vi "_PC_Pub_FM ctrlInstrRefNum.vi"(7 "function":T1, 8 "error in (no error)":errorcluster, 11 "Refnum":T2) -> (0 "error out":errorcluster)   [LabVIEW 2018]
uses:
  ctl/_PC_Pub_FM ctrlFileRefnumEnum.ctl
  Constant/AccessFolderName.ctl
  Ctl/RegistyFunc.ctl
  ctl/_PC_Pub_FM stateMachineEnum.ctl
  <vilib>/Utility/error.llb/Error Cluster From Error Code.vi
  <vilib>/ErrorRing/Error Ring.xnode
  FM.lvclass
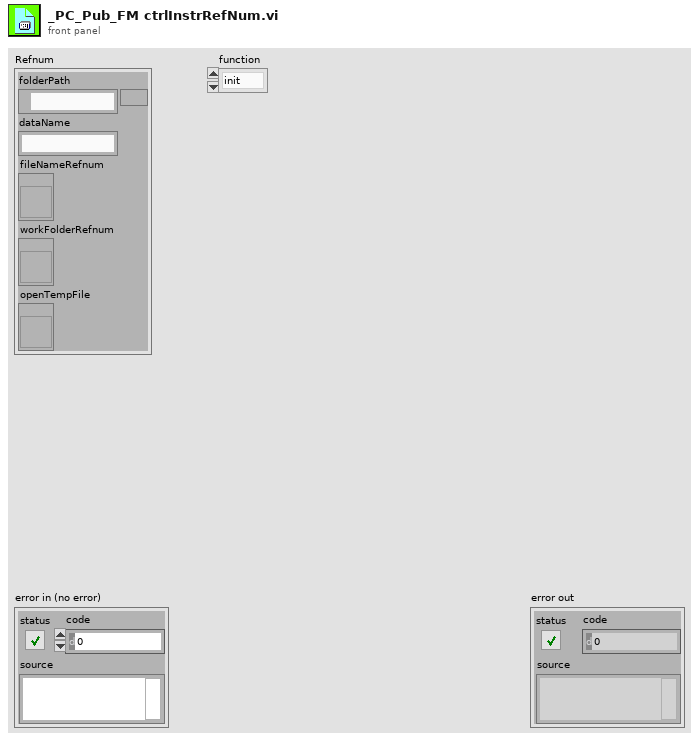
[diagram p1: front panel]
types:
  T1 = typedef "_PC_Pub_FM ctrlFileRefnumEnum.ctl" = enum16{"init", "checkFileName", "updFileName", "updWorkFolder", "updDataItems", "addNewFileName", "addSerialNum"}
  T2 = cluster{"folderPath":path, "dataName":string, "fileNameRefnum":refnum<vi>, "workFolderRefnum":refnum<vi>, "openTempFile":refnum<vi>}
  T3 = typedef "_PC_Pub_FM stateMachineEnum.ctl" = enum16{"none", "init", "reset_t0", "openTDMS", "writeTDMS", "closeTDMS", "readTDMS", "getDataItems"}
  T4 = typedef "RegistyFunc.ctl" = enum16{"None", "FileAutoSave", "FileNoise", "FileSN", "ExeStatu", "WorkFolderPath", "MethodPath", "AVGItem", "LoopItem", "AutoRun", "BGColor", "LineColor", "LineWidth", "XGrid", "YGrid", "DeviceRefnum"}
  T5 = typedef "AccessFolderName.ctl" = enum16{"None", "system_log", "ui_log", "msdata", "method", "d999_param"}
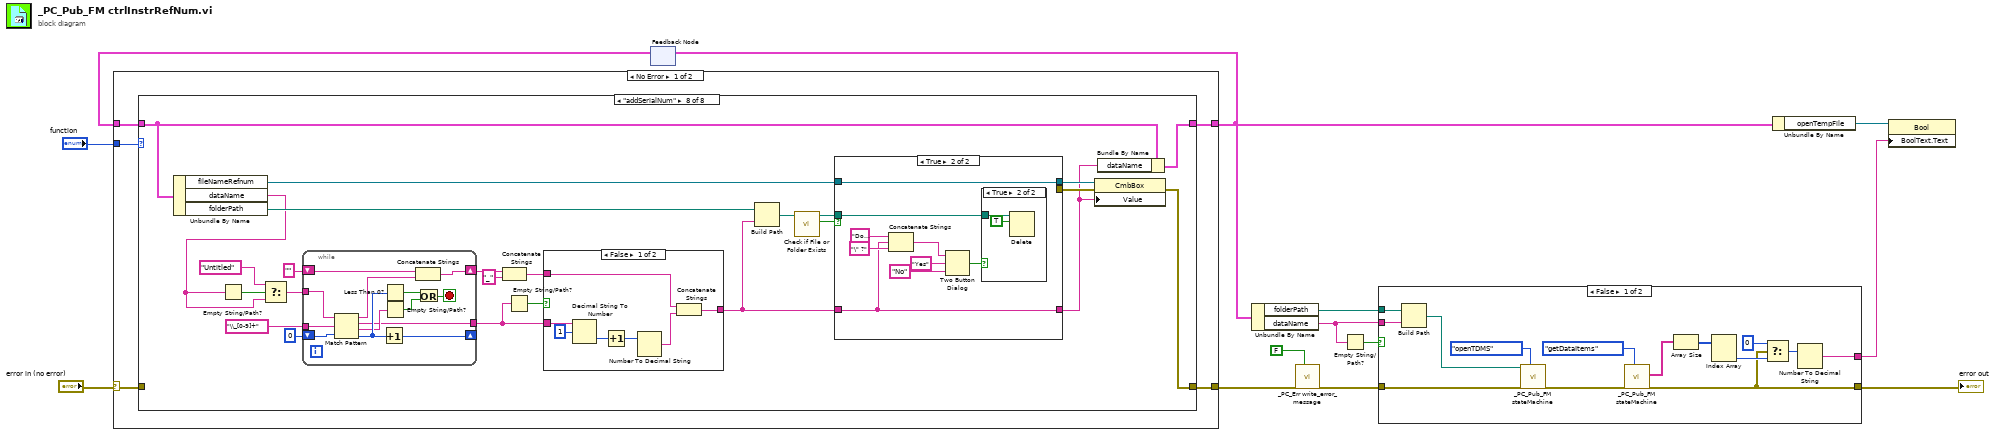
[diagram p0: block diagram]
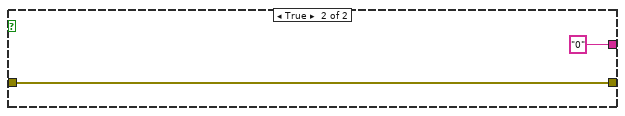
[diagram p2: hidden frame]
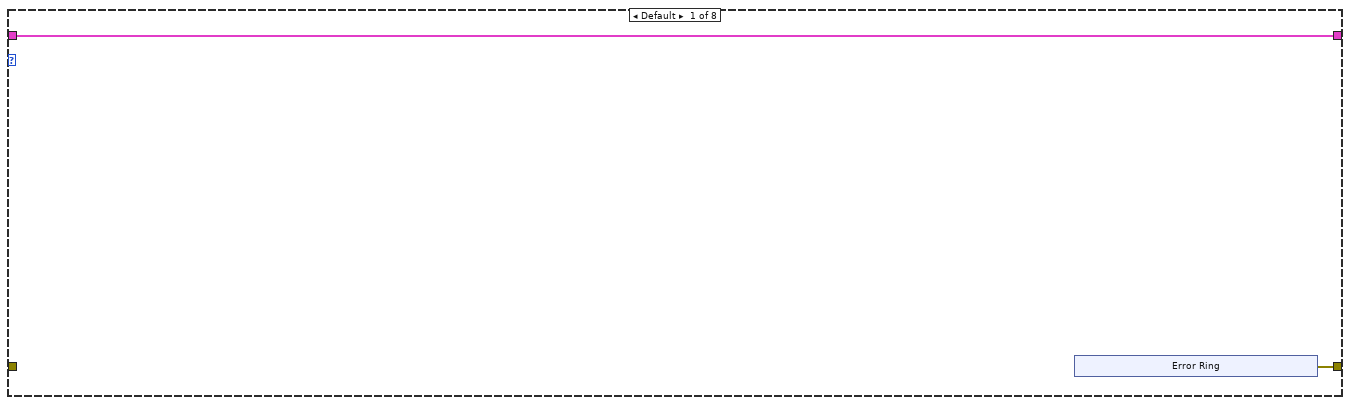
[diagram p3: hidden frame]
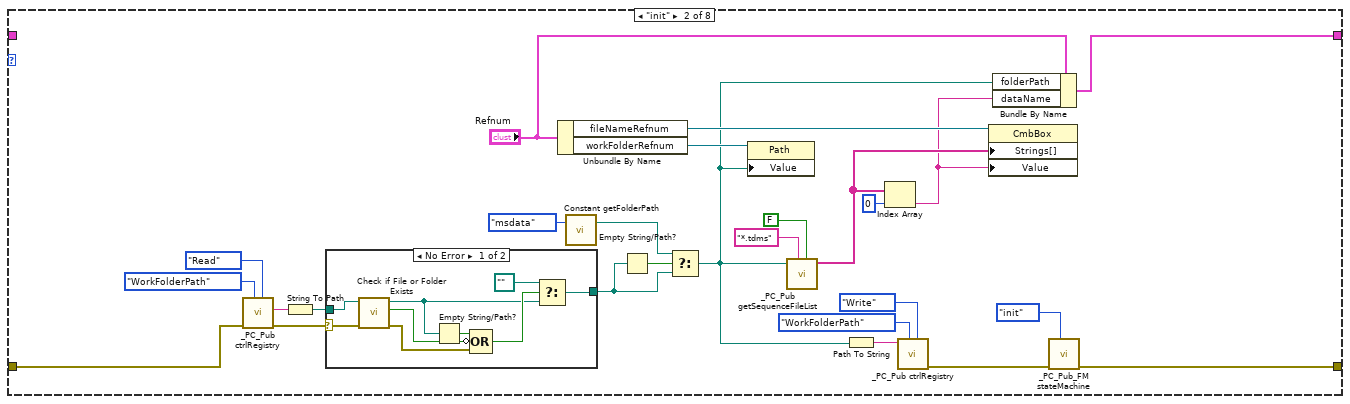
[diagram p4: hidden frame]
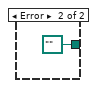
[diagram p5: hidden frame]
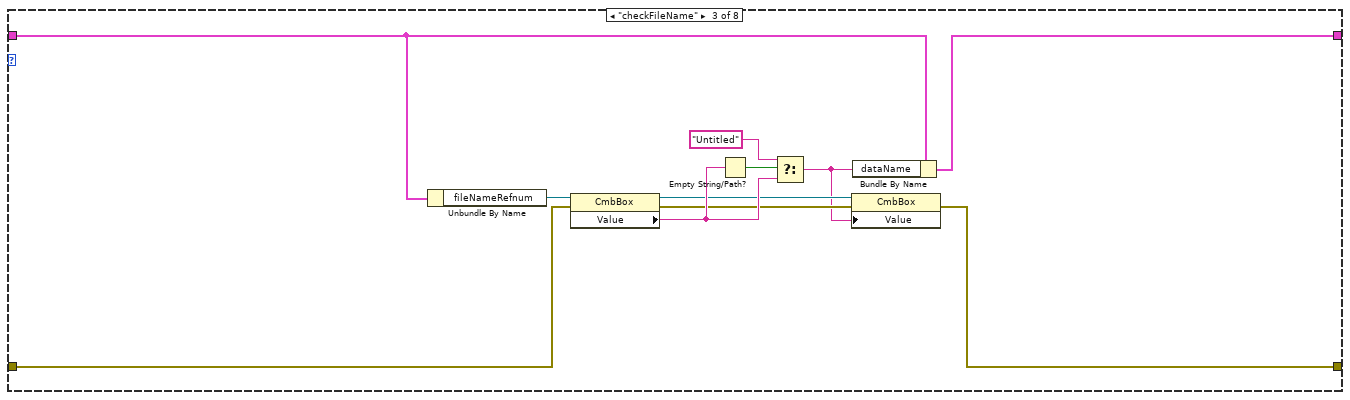
[diagram p6: hidden frame]
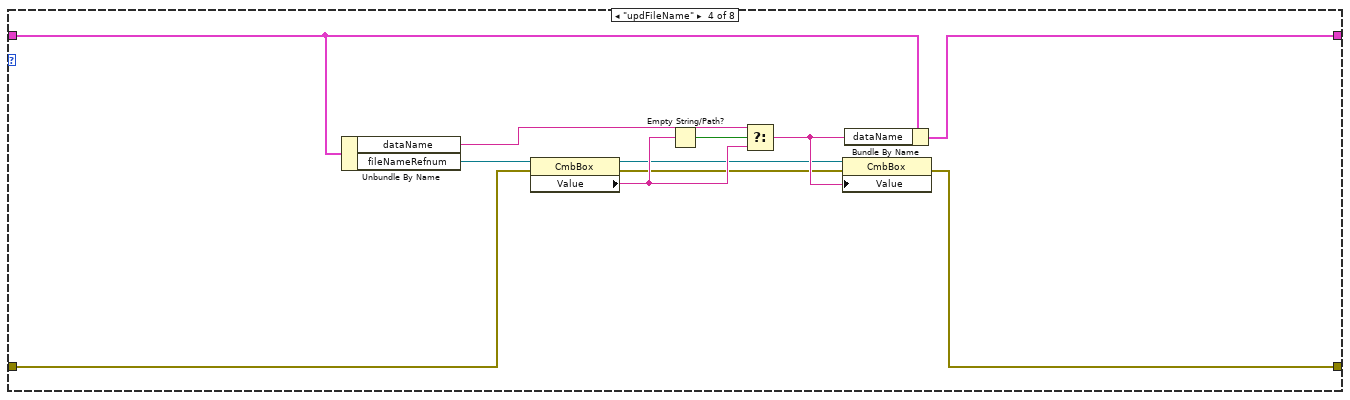
[diagram p7: hidden frame]
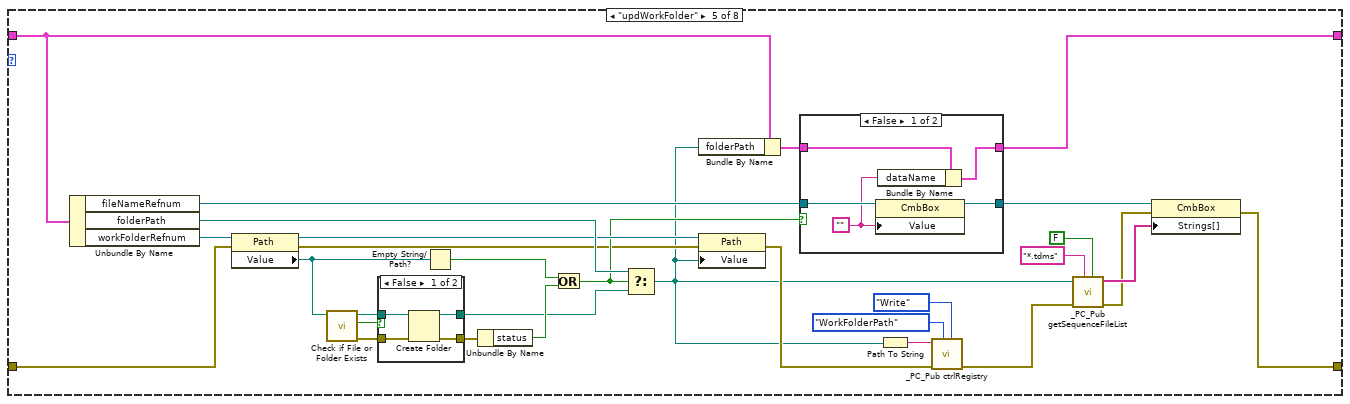
[diagram p8: hidden frame]
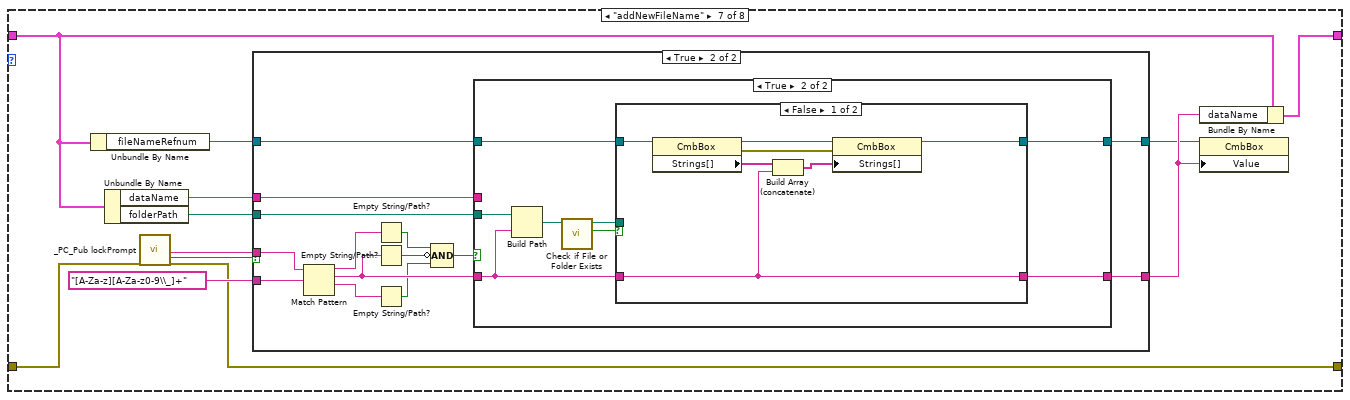
[diagram p12: hidden frame]
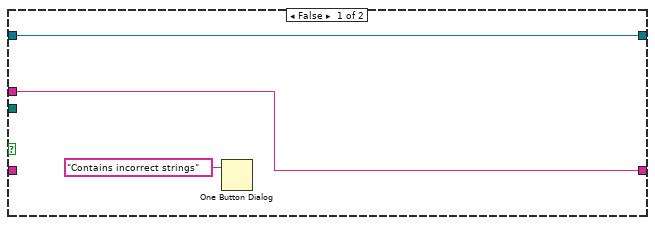
[diagram p14: hidden frame]
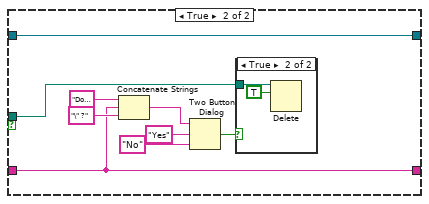
[diagram p15: hidden frame]
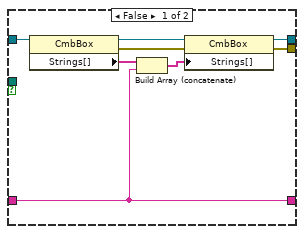
[diagram p17: hidden frame]
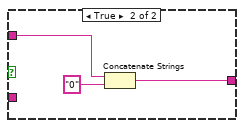
[diagram p19: hidden frame]
diagram:
  n1 = feedback #1() -> (w12:T2)  [unwired: 1 in]
  n2 = case shown="No Error" "error in (no error)" {
    selector: "error in (no error)" -> [w14 w251]
    tunnel: "function" -> [w18 _]
    tunnel: w12 -> [w17 w252]
    tunnel: [w16 w252] -> w7
    tunnel: [w15 w251] -> w8
    frame No Error {
      n3 = case shown="\"addSerialNum\"" w18 {
        tunnel: w17 -> [w20 _ w67 w82 w101 w127 w130 w208]
        tunnel: [w20 w37 w63 w80 w98 w127 w134 w207] -> w16
        tunnel: [w19 w27 w61 w72 w83 w126 w133 w190] -> w15
        tunnel: w14 -> [_ w30 w62 w73 w107 w126 w132 _]
        frame Default {
          n4 = xnode "Error Ring"() -> ("error out"=w19:errorcluster)
        }
        frame "init" {
          n5 = call "_PC_Pub ctrlRegistry.vi"("type"=enum16{"None", "Write", "Read"}."Read", "function"=RegistyFunc."WorkFolderPath", "error in (no error)"=w30) -> ("error out"=w47:errorcluster, "SZ output"=w48:string)  [unwired: 5 in, 2 out]
          n6 = String To Path(string=w48) -> (path=w46:path)
          n7 = case shown="No Error" w47 {
            selector: w47 -> [w58 _]
            tunnel: w46 -> [w59 _]
            tunnel: [w51 path "" ("dup path")] -> w43
            frame No Error {
              n8 = call <vilib>:"Check if File or Folder Exists.vi"("error in (no error)"=w58, "path"=w59) -> ("error out"=w55:errorcluster, "file or folder exists?"=w56:bool, "dup path"=w52:path)  [unwired: 7 in]
              n9 = Empty String/Path?(string/path=w52) -> (empty?=w57:bool)
              n10 = Compound Arithmetic op=OR(w57, invert w56, w55) -> (w54:bool)
              n11 = Select(t=path "" ("dup path"), s=w54, f=w52) -> (s? t:f=w51:path)
            }
            frame Error {
            }
          }
          n12 = Unbundle By Name("Refnum") -> ("fileNameRefnum"=w36:refnum<vi>, "workFolderRefnum"=w39:refnum<vi>)
          n13 = call "Constant getFolderPath.vi"("folder name"=AccessFolderName."msdata") -> ("folder path"=w42:path)  [unwired: 1 in, 1 out]
          n14 = Empty String/Path?(string/path=w43) -> (empty?=w44:bool)
          n15 = Select(t=w42, s=w44, f=w43) -> (s? t:f=w31:path)
          n16 = property class="Path"(reference=w39, "Value"=w31) -> ()  [unwired: 1 in, 2 out]
          n17 = call "_PC_Pub getSequenceFileList.vi"("extention name? (T)"=FALSE, "pattern"="*.tdms", "folderPath"=w31) -> ("listDataName"=w35:string[])  [unwired: 7 in, 1 out]
          n18 = Path To String(path=w31) -> (string=w32:string)
          n19 = Index Array(array=w35, index=0) -> (element=w25:string)
          n20 = call "_PC_Pub ctrlRegistry.vi"("type"=enum16{"None", "Write", "Read"}."Write", "function"=RegistyFunc."WorkFolderPath", "write value"=w32) -> ("error out"=w28:errorcluster)  [unwired: 5 in, 3 out]
          n21 = property class="CmbBox"(reference=w36, "Strings[]"=w35, "Value"=w25) -> ()  [unwired: 1 in, 2 out]
          n22 = Bundle By Name(cluster="Refnum", "folderPath"=w31, "dataName"=w25) -> (w37:T2)
          n23 = call "_PC_Pub_FM stateMachine.vi"("Func"=_PC_Pub_FM_stateMachineEnum."init", "error in (no error)"=w28) -> ("error out"=w27:errorcluster)  [unwired: 7 in, 2 out]
        }
        frame "checkFileName" {
          n24 = Unbundle By Name(w67) -> ("fileNameRefnum"=w71:refnum<vi>)
          n25 = property class="CmbBox"(reference=w71, error in=w62) -> (reference out=w66:refnum<vi>, error out=w65:errorcluster, "Value"=w69:string)
          n26 = Empty String/Path?(string/path=w69) -> (empty?=w70:bool)
          n27 = Select(t="Untitled", s=w70, f=w69) -> (s? t:f=w64:string)
          n28 = property class="CmbBox"(reference=w66, error in=w65, "Value"=w64) -> (error out=w61:errorcluster)  [unwired: 1 out]
          n29 = Bundle By Name(cluster=w67, "dataName"=w64) -> (w63:T2)
        }
        frame "updFileName" {
          n30 = Unbundle By Name(w82) -> ("dataName"=w78:string, "fileNameRefnum"=w76:refnum<vi>)
          n31 = property class="CmbBox"(reference=w76, error in=w73) -> (reference out=w75:refnum<vi>, error out=w74:errorcluster, "Value"=w77:string)
          n32 = Empty String/Path?(string/path=w77) -> (empty?=w79:bool)
          n33 = Select(t=w78, s=w79, f=w77) -> (s? t:f=w81:string)
          n34 = property class="CmbBox"(reference=w75, error in=w74, "Value"=w81) -> (error out=w72:errorcluster)  [unwired: 1 out]
          n35 = Bundle By Name(cluster=w82, "dataName"=w81) -> (w80:T2)
        }
        frame "updWorkFolder" {
          n36 = Unbundle By Name(w101) -> ("fileNameRefnum"=w99:refnum<vi>, "folderPath"=w109:path, "workFolderRefnum"=w108:refnum<vi>)
          n37 = property class="Path"(reference=w108, error in=w107) -> (reference out=w106:refnum<vi>, error out=w89:errorcluster, "Value"=w97:path)
          n38 = call <vilib>:"Check if File or Folder Exists.vi"("path"=w97) -> ("error out"=w110:errorcluster, "file or folder exists?"=w112:bool, "dup path"=w111:path)  [unwired: 8 in]
          n39 = case shown="False" w112 {
            tunnel: w111 -> [w123 w124]
            tunnel: w110 -> [w122 w125]
            tunnel: [w121 w124] -> w93
            tunnel: [w120 w125] -> w96
            frame False {
              n40 = Create Folder(path (use dialog)=w123, error in=w122) -> (created path=w121:path, error out=w120:errorcluster)  [unwired: 1 in, 1 out]
            }
            frame True {
            }
          }
          n41 = Empty String/Path?(string/path=w97) -> (empty?=w95:bool)
          n42 = Unbundle By Name(w96) -> ("status"=w94:bool)
          n43 = Or(x=w95, y=w94) -> (x .or. y?=w92:bool)
          n44 = Select(t=w109, s=w92, f=w93) -> (s? t:f=w88:path)
          n45 = Bundle By Name(cluster=w101, "folderPath"=w88) -> (w100:T2)
          n46 = property class="Path"(reference=w106, error in=w89, "Value"=w88) -> (error out=w102:errorcluster)  [unwired: 1 out]
          n47 = case shown="False" w92 {
            tunnel: w100 -> [w116 w119]
            tunnel: w99 -> [w117 w118]
            tunnel: [w114 w119] -> w98
            tunnel: [w113 w118] -> w86
            frame False {
              w115 = ""
              n48 = property class="CmbBox"(reference=w117, "Value"=w115) -> (reference out=w113:refnum<vi>)  [unwired: 1 in, 1 out]
              n49 = Bundle By Name(cluster=w116, "dataName"=w115) -> (w114:T2)
            }
            frame True {
            }
          }
          n50 = Path To String(path=w88) -> (string=w103:string)
          n51 = call "_PC_Pub ctrlRegistry.vi"("type"=enum16{"None", "Write", "Read"}."Write", "function"=RegistyFunc."WorkFolderPath", "error in (no error)"=w102, "write value"=w103) -> ("error out"=w87:errorcluster)  [unwired: 4 in, 3 out]
          n52 = call "_PC_Pub getSequenceFileList.vi"("extention name? (T)"=FALSE, "pattern"="*.tdms", "error in (no error)"=w87, "folderPath"=w88) -> ("error out"=w84:errorcluster, "listDataName"=w85:string[])  [unwired: 6 in]
          n53 = property class="CmbBox"(reference=w86, error in=w84, "Strings[]"=w85) -> (error out=w83:errorcluster)  [unwired: 1 out]
        }
        frame "updDataItems" {
        }
        frame "addNewFileName" {
          n54 = Unbundle By Name(w130) -> ("fileNameRefnum"=w128:refnum<vi>)
          n55 = Unbundle By Name(w130) -> ("dataName"=w136:string, "folderPath"=w131:path)
          n56 = call "_PC_Pub lockPrompt.vi"("error in (no error)"=w132) -> ("New Group Name"=w138:string, "OK"=w139:bool, "error out"=w133:errorcluster)  [unwired: 16 in]
          n57 = case shown="True" w139 {
            tunnel: w138 -> [_ w155]
            tunnel: "[A-Za-z][A-Za-z0-9\\_]+" ("regular expression") -> [_ w154]
            tunnel: [w141 w151] -> w135
            tunnel: w136 -> [w141 w150]
            tunnel: w131 -> [_ w149]
            tunnel: [w140 w148] -> w129
            tunnel: w128 -> [w140 w147]
            frame False {
            }
            frame True {
              n58 = Match Pattern(string=w155, regular expression=w154) -> (before substring=w153:string, match substring=w146:string, after substring=w152:string)  [unwired: 1 in, 1 out]
              n59 = Empty String/Path?(string/path=w153) -> (empty?=w145:bool)
              n60 = Empty String/Path?(string/path=w146) -> (empty?=w144:bool)
              n61 = Empty String/Path?(string/path=w152) -> (empty?=w143:bool)
              n62 = Compound Arithmetic op=AND(w145, invert w144, w143) -> (w142:bool)
              n63 = case shown="True" w142 {
                tunnel: w146 -> [_ w165]
                tunnel: [w157 w162] -> w151
                tunnel: w150 -> [w157 _]
                tunnel: w149 -> [_ w166]
                tunnel: [w156 w161] -> w148
                tunnel: w147 -> [w156 w160]
                frame False {
                  n64 = One Button Dialog(message="Contains incorrect strings") -> ()  [unwired: 1 in, 1 out]
                }
                frame True {
                  n65 = Build Path(base path=w166, name or relative path=w165) -> (appended path=w164:path)
                  n66 = call <vilib>:"Check if File or Folder Exists.vi"("path"=w164) -> ("file or folder exists?"=w163:bool, "dup path"=w159:path)  [unwired: 8 in, 1 out]
                  n67 = case shown="False" w163 {
                    tunnel: w165 -> [w169 w175]
                    tunnel: [w169 w175] -> w162
                    tunnel: [w167 w182] -> w161
                    tunnel: w160 -> [w168 w182]
                    tunnel: w159 -> [_ w174]
                    frame False {
                      n68 = property class="CmbBox"(reference=w168) -> (reference out=w172:refnum<vi>, error out=w171:errorcluster, "Strings[]"=w173:string[])  [unwired: 1 in]
                      n69 = Build Array (concatenate)(w173, w169) -> (w170:string[])
                      n70 = property class="CmbBox"(reference=w172, error in=w171, "Strings[]"=w170) -> (reference out=w167:refnum<vi>)  [unwired: 1 out]
                    }
                    frame True {
                      n71 = Concatenate Strings("Do you want to overwrite \"" ("message"), w175, "\" ?" ("message")) -> (w180:string)
                      n72 = Two Button Dialog(message=w180, 1:"No" ("F button name (\"Cancel\")"), 2:"Yes" ("T button name (\"OK\")")) -> (T button?=w181:bool)
                      n73 = case shown="True" w181 {
                        tunnel: w174 -> [_ w184]
                        frame False {
                        }
                        frame True {
                          n74 = Delete(path (use dialog)=w184, entire hierarchy (F)=TRUE) -> ()  [unwired: 3 in, 3 out]
                        }
                      }
                    }
                  }
                }
              }
            }
          }
          n75 = Bundle By Name(cluster=w130, "dataName"=w135) -> (w134:T2)
          n76 = property class="CmbBox"(reference=w129, "Value"=w135) -> ()  [unwired: 1 in, 2 out]
        }
        frame "addSerialNum" {
          n77 = Unbundle By Name(w208) -> ("fileNameRefnum"=w198:refnum<vi>, "dataName"=w185:string, "folderPath"=w196:path)
          n78 = Empty String/Path?(string/path=w185) -> (empty?=w188:bool)
          n79 = Select(t="Untitled", s=w188, f=w185) -> (s? t:f=w186:string)
          n80 = while {
            tunnel: w186 -> [w249]
            tunnel: "\\_[0-9]+" ("regular expression") -> [w250]
            shift-right: [w247] -> _
            shift-left: 0 -> [w248]
            tunnel: [w241] -> w202
            shift-right: [w238] -> w201
            shift-left: "" -> [w240]
            stop <- w242 stop-if-true
            n81 = Match Pattern(string=w249, regular expression=w250, offset (0)=w248) -> (before substring=w239:string, match substring=w241:string, after substring=w245:string, offset past match=w246:i32)
            n82 = Increment(x=w246) -> (x+1=w247:i32)
            n83 = Less Than 0?(x=w246) -> (x < 0?=w244:bool)
            n84 = Empty String/Path?(string/path=w245) -> (empty?=w243:bool)
            n85 = Concatenate Strings(w240, w239) -> (w238:string)
            n86 = Or(x=w244, y=w243) -> (x .or. y?=w242:bool)
          }
          n87 = Concatenate Strings(w201, "_" ("string")) -> (w199:string)
          n88 = Empty String/Path?(string/path=w202) -> (empty?=w203:bool)
          n89 = case shown="False" w203 {
            tunnel: w199 -> [w230 w237]
            tunnel: w202 -> [w233 _]
            tunnel: [w228 w235] -> w195
            frame False {
              n90 = Decimal String To Number(string=w233, offset=1) -> (number=w232:i32)  [unwired: 1 in, 1 out]
              n91 = Increment(x=w232) -> (x+1=w231:i32)
              n92 = Number To Decimal String(number=w231) -> (decimal integer string=w229:string)  [unwired: 1 in]
              n93 = Concatenate Strings(w230, w229) -> (w228:string)
            }
            frame True {
              n94 = Concatenate Strings(w237, "0" ("string")) -> (w235:string)
            }
          }
          n95 = Build Path(base path=w196, name or relative path=w195) -> (appended path=w197:path)
          n96 = call <vilib>:"Check if File or Folder Exists.vi"("path"=w197) -> ("file or folder exists?"=w194:bool, "dup path"=w189:path)  [unwired: 8 in, 1 out]
          n97 = case shown="True" w194 {
            tunnel: w198 -> [w216 w225]
            tunnel: [w211 _] -> w192
            tunnel: w195 -> [w209 w222]
            tunnel: [w209 w222] -> w191
            tunnel: [w210 w225] -> w193
            tunnel: w189 -> [_ w217]
            frame False {
              n98 = property class="CmbBox"(reference=w216) -> (reference out=w214:refnum<vi>, error out=w213:errorcluster, "Strings[]"=w215:string[])  [unwired: 1 in]
              n99 = Build Array (concatenate)(w215, w209) -> (w212:string[])
              n100 = property class="CmbBox"(reference=w214, error in=w213, "Strings[]"=w212) -> (reference out=w210:refnum<vi>, error out=w211:errorcluster)
            }
            frame True {
              n101 = Concatenate Strings("Do you want to overwrite \"" ("message"), w222, "\" ?" ("message")) -> (w219:string)
              n102 = Two Button Dialog(message=w219, 1:"No" ("F button name (\"Cancel\")"), 2:"Yes" ("T button name (\"OK\")")) -> (T button?=w218:bool)
              n103 = case shown="True" w218 {
                tunnel: w217 -> [_ w227]
                frame False {
                }
                frame True {
                  n104 = Delete(path (use dialog)=w227, entire hierarchy (F)=TRUE) -> ()  [unwired: 3 in, 3 out]
                }
              }
            }
          }
          n105 = property class="CmbBox"(reference=w193, error in=w192, "Value"=w191) -> (error out=w190:errorcluster)  [unwired: 1 out]
          n106 = Bundle By Name(cluster=w208, "dataName"=w191) -> (w207:T2)
        }
      }
    }
    frame Error {
    }
  }
  n107 = feedback-in #1(w7) -> ()
  n108 = Unbundle By Name(w7) -> ("folderPath"=w6:path, "dataName"=w5:string)
  n109 = call "_PC_Err write_error_message.vi"("show msg( T )"=FALSE, "error in"=w8) -> ("error out"=w2:errorcluster)  [unwired: 9 in]
  n110 = Empty String/Path?(string/path=w5) -> (empty?=w4:bool)
  n111 = case shown="False" w4 {
    tunnel: [w263 "0"] -> w10
    tunnel: w6 -> [w261 _]
    tunnel: w5 -> [w260 _]
    tunnel: w2 -> [w254 w267]
    tunnel: [w253 w267] -> w1
    frame False {
      n112 = Build Path(base path=w261, name or relative path=w260) -> (appended path=w258:path)
      n113 = call "_PC_Pub_FM stateMachine.vi"("Func"=_PC_Pub_FM_stateMachineEnum."openTDMS", "error in (no error)"=w254, "tdmsFilePath in"=w258) -> ("error out"=w256:errorcluster)  [unwired: 6 in, 2 out]
      n114 = call "_PC_Pub_FM stateMachine.vi"("Func"=_PC_Pub_FM_stateMachineEnum."getDataItems", "error in (no error)"=w256) -> ("error out"=w253:errorcluster, "outputDataArray"=w255:string[][])  [unwired: 7 in, 1 out]
      n115 = Array Size(array=w255) -> (size(s)=w266:i32[])
      n116 = Index Array(array=w266) -> (element #2=w262:i32)  [unwired: 2 in, 1 out]
      n117 = Select(t=0, s=w253, f=w262) -> (s? t:f=w264:i32)
      n118 = Number To Decimal String(number=w264) -> (decimal integer string=w263:string)  [unwired: 1 in]
    }
    frame True {
    }
  }
  "error out" <- w1
  n119 = Unbundle By Name(w7) -> ("openTempFile"=w11:refnum<vi>)
  n120 = property class="Bool"(reference=w11, "BoolText.Text"=w10) -> ()  [unwired: 1 in, 2 out]
